vi "Array has been Searched for Signed Integers.vi"(11 "JSON Parser in":refnum<class "JSON Parser.lvclass">) -> (3 "JSON Parser out":refnum<class "JSON Parser.lvclass">)   [LabVIEW 2020, in "JKI JSON Serialization.lvlib" / "JSON Parser.lvclass"]
uses:
  JSON Parser.lvclass
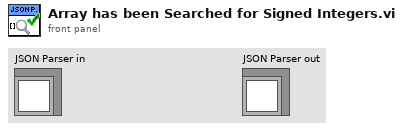
[diagram p1: front panel]
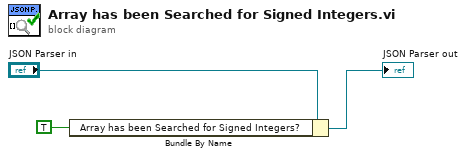
[diagram p0: block diagram]
diagram:
  n1 = Bundle By Name(cluster="JSON Parser in", "Array has been Searched for Signed Integers?"=TRUE) -> (→"JSON Parser out":refnum<class "JSON Parser.lvclass">)
